vi "PixyCamSPI.vi"(11 "SPI Bus":T1) -> ()   [LabVIEW 2016]
doc: "This VI reads the bolcks identified by a PixyCam. It is designed within the FRC framework and is expected to be run on a RoboRIO using the SPI ports.\nThe slave select pins are used so several PixyCam can be used. \nRefer to http://cmucam.org/projects/cmucam5/wiki/Porting_Guide for wiring and code explanation\nUse PixyMon to define the protocol and signatures\n\n(c)2017 PY Le Bas"
uses:
  <vilib>/Rock Robotics/SystemInterfaces/spilib/spi_bus.ctl
  <vilib>/Rock Robotics/WPI/SPI/WPI_SPIMode.ctl
  Robot Global Data.vi
  <vilib>/Rock Robotics/Network Tables/NT Write Number.vi
panel:
  in  "MinSize":u16=10
  out "Blocks":T2(array[cluster])
  out "last frame data":u16[](array[numeric]) format="%.0x"
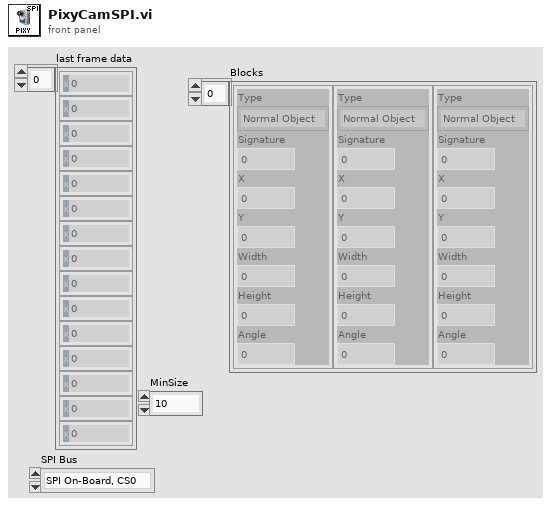
[diagram p1: front panel]
types:
  T1 = typedef "spi_bus.ctl" = enum16{"SPI On-Board, CS0", "SPI On-Board, CS1", "SPI On-Board, CS2", "SPI On-Board, CS3", "SPI MXP", "Invalid"}
  T2 = cluster{"Type":enum16{"Normal Object", "Color Object"}, "Signature":u16, "X":u16, "Y":u16, "Width":u16, "Height":u16, "Angle":u16}[]
  T3 = typedef "WPI_SPIMode.ctl" = enum16{"Mode 0 (Clk Idle Low,Sample on Leading)", "Mode 1 (Clk Idle Low,Sample on Trailing)", "Mode 2 (Clk Idle High,Sample on Leading)", "Mode 3 (Clk Idle High,Sample on Trailing)"}
  T4 = typedef "WPI_SPIDevRef.ctl" = cluster{"DevStatus":errorcluster, "Handle":i32, "SPI Bus":T1}
  T5 = typedef "WPI_DriverStationRobotMode2.ctl" = enum16{"Autonomous Disabled", "Autonomous Enabled", "Teleop Disabled", "Teleop Enabled", "Disconnected", "Finish", "Test Disabled", "Test Enabled", "Emergency Stopped"}
  T6 = cluster{"Type":enum16{"Normal Object", "Color Object"}, "Signature":u16, "X":u16, "Y":u16, "Width":u16, "Height":u16, "Angle":u16}
  T7 = cluster{"[0]":u16, "[1]":u16, "[2]":u16, "[3]":u16, "[4]":u16, "[5]":u16, "[6]":u16}
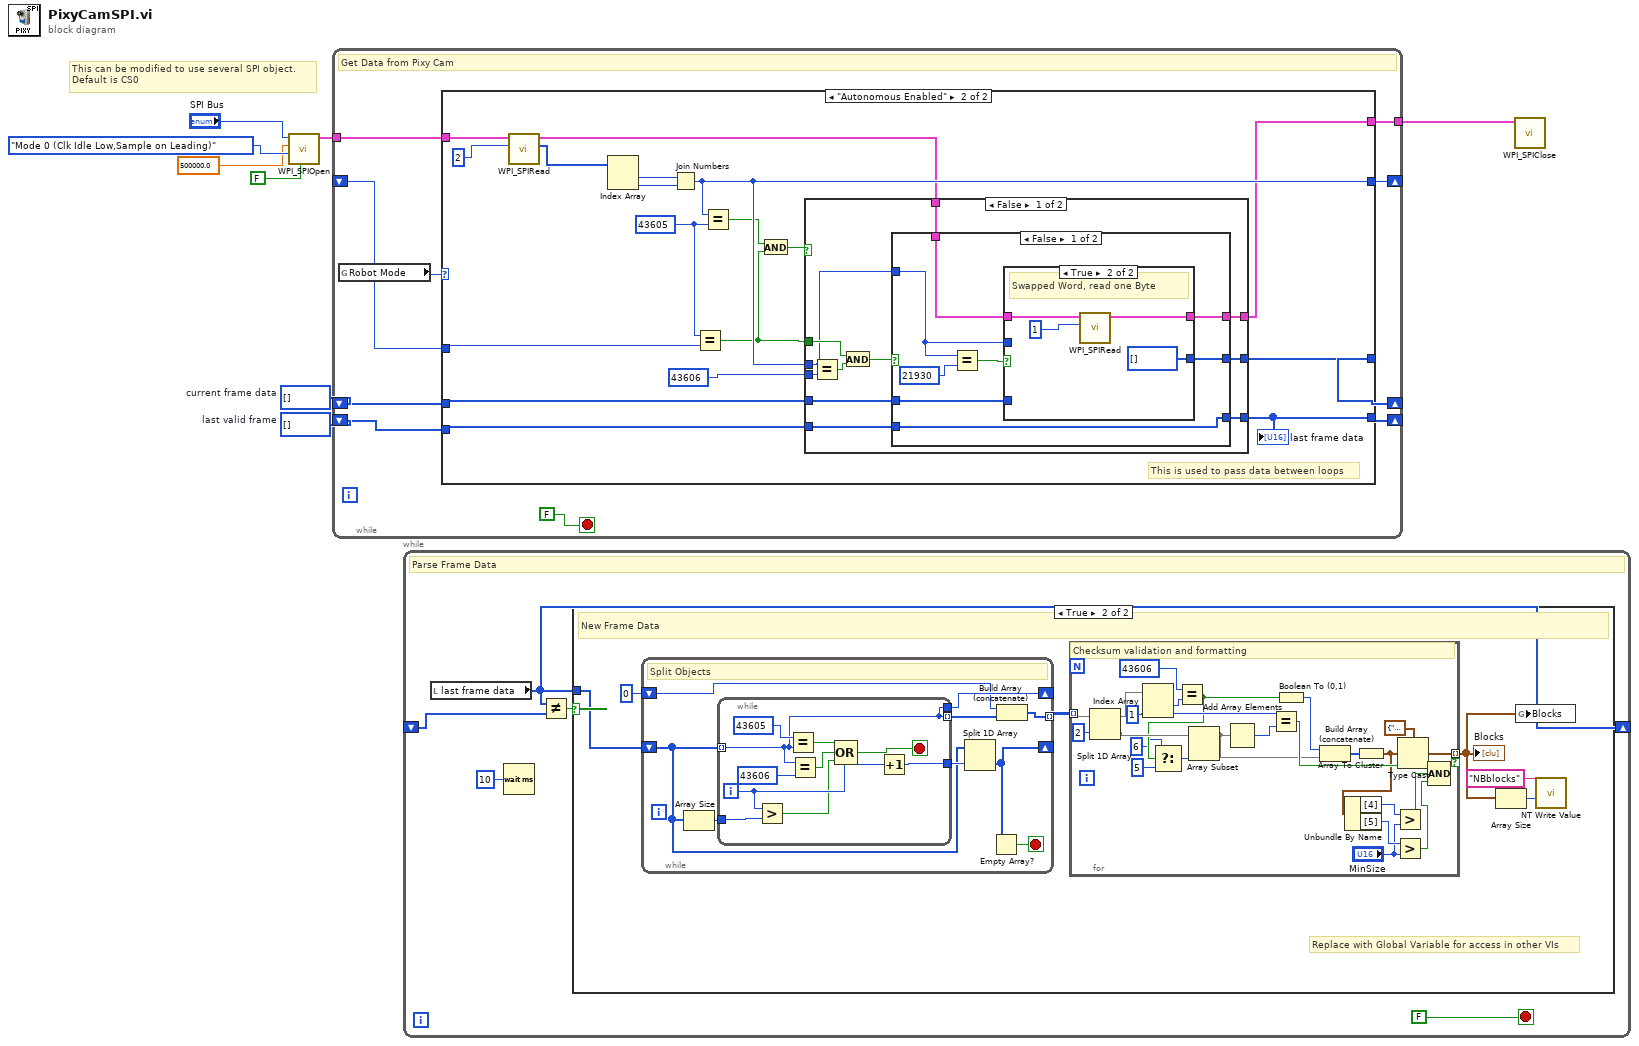
[diagram p0: block diagram]
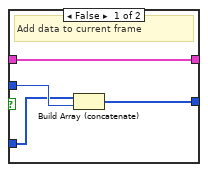
[diagram p4: hidden frame]
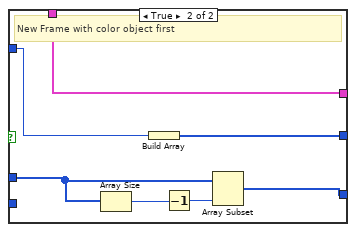
[diagram p5: hidden frame]
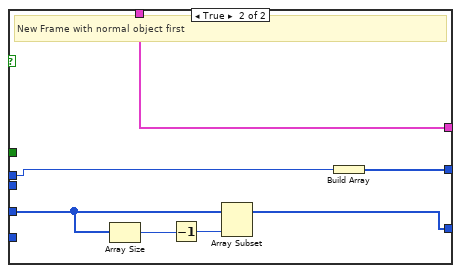
[diagram p6: hidden frame]
diagram:
  w5 = u16[] []  # current frame data
  w6 = u16[] []  # last valid frame
  # "This can be modified to use several SPI object.\nDefault is CS0"
  n1 = call <vilib>:"WPI_SPIOpen.vi"("Chip Select Active High (F)"=FALSE, "Mode (3)"=WPI_SPIMode."Mode 0 (Clk Idle Low,Sample on Leading)", "Clock Rate (Hz)"=500000.0, "SPI Bus"="SPI Bus") -> ("SPIDevRef"=w8:T4)  [unwired: 6 in, 1 out]
  n2 = while {
    tunnel: w8 -> [w18]
    tunnel: [w15] -> w7
    shift-right: [w16] -> _
    shift-left: _ -> [w17]
    shift-right: [w13] -> _
    shift-left: w5 -> [w14]
    shift-right: [w12] -> _
    shift-left: w6 -> [w11]
    stop <- FALSE stop-if-true
    # "Get Data from Pixy Cam"
    n3 = global read "Robot Global Data.vi" "Robot Mode"() -> (w9:T5)
    n4 = case shown="\"Autonomous Enabled\"" w9 {
      tunnel: w18 -> [w22 w40]
      tunnel: w17 -> [w21 w39]
      tunnel: [w21 w38] -> w16
      tunnel: [w22 w37] -> w15
      tunnel: w14 -> [w20 w36]
      tunnel: [w20 w35] -> w13
      tunnel: [w19 w34] -> w12
      tunnel: w11 -> [w19 w33]
      frame "Autonomous Disabled", Default {
      }
      frame "Autonomous Enabled" {
        w24 = u16 43605
        # "This is used to pass data between loops"
        n5 = call <vilib>:"WPI_SPIRead.vi"("Num to Read"=2, "SPIDevRef"=w40) -> ("Received Data"=w32:u8[], "SPIDevRef"=w25:T4)  [unwired: 7 in, 1 out]
        n6 = Index Array(array=w32) -> (element #1=w31:u8, element #2=w30:u8)  [unwired: 2 in]
        n7 = Join Numbers(hi=w31, lo=w30) -> ((hi.lo)=w38:u16)
        n8 = Equal?(x=w24, y=w39) -> (x = y?=w27:bool)
        n9 = Equal?(x=w38, y=w24) -> (x = y?=w28:bool)
        n10 = And(x=w28, y=w27) -> (x .and. y?=w29:bool)
        n11 = case shown="False" w29 {
          tunnel: w27 -> [w51 _]
          tunnel: w38 -> [w41 w75]
          tunnel: u16 43606 -> [w49 _]
          tunnel: w25 -> [w47 w81]
          tunnel: [w46 w81] -> w37
          tunnel: w36 -> [w45 w78]
          tunnel: [w44 w76] -> w35
          tunnel: [w43 w80] -> w34
          tunnel: w33 -> [w42 _]
          frame False {
            n12 = Equal?(x=w41, y=w49) -> (x = y?=w50:bool)
            n13 = And(x=w51, y=w50) -> (x .and. y?=w48:bool)
            n14 = case shown="False" w48 {
              tunnel: w41 -> [w55 w69]
              tunnel: w47 -> [w58 w74]
              tunnel: [w57 w74] -> w46
              tunnel: w45 -> [w54 w71]
              tunnel: [w53 w68] -> w44
              tunnel: [w52 w70] -> w43
              tunnel: w42 -> [w52 _]
              frame False {
                n15 = Equal?(x=w55, y=u16 21930) -> (x = y?=w56:bool)
                n16 = case shown="True" w56 {
                  tunnel: w58 -> [w63 w67]
                  tunnel: [w63 w66] -> w57
                  tunnel: w55 -> [w62 _]
                  tunnel: w54 -> [w61 _]
                  tunnel: [w60 u16[] []] -> w53
                  frame False {
                    # "Add data to current frame"
                    n17 = Build Array (concatenate)(w61, w62) -> (w60:u16[])
                  }
                  frame True {
                    # "Swapped Word, read one Byte"
                    n18 = call <vilib>:"WPI_SPIRead.vi"("Num to Read"=1, "SPIDevRef"=w67) -> ("SPIDevRef"=w66:T4)  [unwired: 7 in, 2 out]
                  }
                }
              }
              frame True {
                # "New Frame with color object first"
                n19 = Array Size(array=w71) -> (size(s)=w73:i32)
                n20 = Build Array(w69) -> (w68:u16[])
                n21 = Decrement(x=w73) -> (x-1=w72:i32)
                n22 = Array Subset(array=w71, length=w72) -> (w70:u16[])  [unwired: 1 in]
              }
            }
          }
          frame True {
            # "New Frame with normal object first"
            n23 = Array Size(array=w78) -> (size(s)=w79:i32)
            n24 = Decrement(x=w79) -> (x-1=w77:i32)
            n25 = Array Subset(array=w78, length=w77) -> (w80:u16[])  [unwired: 1 in]
            n26 = Build Array(w75) -> (w76:u16[])
          }
        }
        "last frame data" <- w34
      }
    }
  }
  n27 = while {
    shift-right: [w84] -> _
    shift-left: _ -> [w86]
    stop <- FALSE stop-if-true
    # "Parse Frame Data"
    n28 = local read "last frame data"() -> (w84:u16[])
    n29 = Wait (ms)(milliseconds to wait=u32 10) -> ()  [unwired: 1 out]
    n30 = Not Equal?(x=w84, y=w86) -> (x != y?=w85:bool)
    n31 = case shown="True" w85 {
      tunnel: w84 -> [_ w91]
      frame False {
        # "Same Frame"
      }
      frame True {
        # "Replace with Global Variable for access in other VIs"
        # "New Frame Data"
        n32 = while {
          shift-right: [w125] -> _
          shift-left: w91 -> [w123]
          tunnel: [w121] -> w90 mode=indexing
          shift-right: [w120] -> _
          shift-left: u16 0 -> [w119]
          stop <- w124 stop-if-true
          # "Split Objects"
          n33 = Array Size(array=w123) -> (size(s)=w122:i32)
          n34 = while {
            tunnel: w123 -> [w128] mode=indexing
            tunnel: [w128] -> w127 mode=indexing
            tunnel: [w133] -> w126
            tunnel: w122 -> [w131]
            tunnel: [w128] -> w120
            i -> [w130]
            stop <- w134 stop-if-true
            n35 = Greater?(x=w130, y=w131) -> (0:w129:bool)
            n36 = Equal?(x=u16 43605, y=w128) -> (x = y?=w136:bool)
            n37 = Equal?(x=w128, y=u16 43606) -> (x = y?=w135:bool)
            n38 = Compound Arithmetic op=OR(w136, w135, w129) -> (w134:bool)
            n39 = Increment(x=w130) -> (x+1=w133:i32)
          }
          n40 = Split 1D Array(array=w123, index=w126) -> (second subarray=w125:u16[])  [unwired: 1 out]
          n41 = Empty Array?(array=w125) -> (empty?=w124:bool)
          n42 = Build Array (concatenate)(w119, w127) -> (w121:u16[])
        }
        n43 = for {
          tunnel: w90 -> [w118] mode=indexing
          tunnel: [w108] -> w87 mode=indexing if=w95
          # "Checksum validation and formatting"
          n44 = Split 1D Array(array=w118, index=2) -> (first subarray=w116:u16[], second subarray=w105:u16[])
          n45 = Index Array(array=w116, index #2=1 ("index")) -> (element #1=w111:u16, element #2=w115:u16)  [unwired: 1 in]
          n46 = Equal?(x=u16 43606, y=w111) -> (x = y?=w102:bool)
          n47 = Select(t=6 ("index"), s=w102, f=5 ("index")) -> (s? t:f=w103:i32)
          n48 = Array Subset(array=w105, length=w103) -> (w104:u16[])  [unwired: 1 in]
          n49 = Add Array Elements(numeric array=w104) -> (sum=w114:u16)
          n50 = Equal?(x=w115, y=w114) -> (x = y?=w106:bool)
          n51 = Boolean To (0,1)(Boolean=w102) -> (0, 1=w109:i16)
          n52 = Build Array (concatenate)(w109, w104) -> (w112:u16[])
          n53 = Array To Cluster(array=w112) -> (cluster=w99:T7)
          n54 = Unbundle By Name(w99) -> ("[4]"=w98:u16, "[5]"=w97:u16)
          n55 = Greater?(x=w98, y="MinSize") -> (0:w93:bool)
          n56 = Greater?(x=w97, y="MinSize") -> (0:w94:bool)
          n57 = Type Cast(type=T6 {"Type"=enum."Color Object", "Signature"=1, "X"=100, "Y"=36, "Width"=50, "Height"=48, "Angle"=0} ("Blocks"), x=w99) -> (*(type *) &x=w108:T6)
          n58 = Compound Arithmetic op=AND(w106, w93, w94) -> (w95:bool)
        }
        "Blocks" <- w87
        n59 = Array Size(array=w87) -> (size(s)=w88:i32)
        n60 = global write "Robot Global Data.vi" "Blocks"(w87) -> ()
        n61 = call-poly <vilib>:"NT Write Value.vi"("Numeric"=w88, "Name"="NBblocks") -> ()  [unwired: 9 in, 1 out]
      }
    }
  }
  n62 = call <vilib>:"WPI_SPIClose.vi"("SPIDevRef"=w7) -> ()  [unwired: 10 in, 1 out]
